vi "action.vi"(0 "HGF_FGV_Index":refnum<class "HGF_FGV_Index.lvclass">, 2 "Objects":refnum<class>[](array[class]), 5 "error in (no error)":errorcluster) -> (14 "dup HGF_FGV_Index":refnum<class "HGF_FGV_Index.lvclass">, 16 "dup Objects":refnum<class>[](array[class]), 19 "error out":errorcluster)   [LabVIEW 2012, in "HGF_FGV.lvlib" / "HGF_FGV_Index.lvclass"]
doc: "Return copy of addressed object from object array."
uses:
  HGF_FGV_Index.lvclass
  HGF_FGV_Index.lvclass/HGF_FGV_Index.ctl
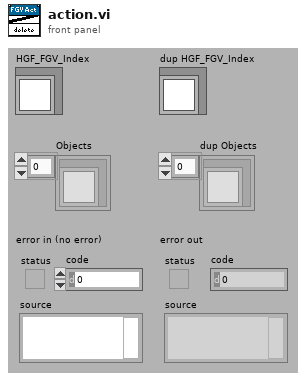
[diagram p1: front panel]
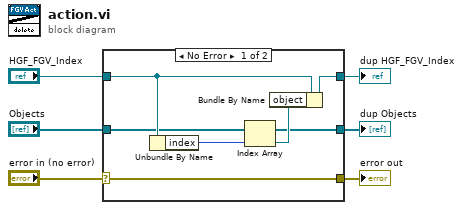
[diagram p0: block diagram]
diagram:
  n1 = case shown="No Error" "error in (no error)" {
    selector: "error in (no error)" -> [w12 w15]
    tunnel: [w12 w15] -> w5
    tunnel: [w11 w14] -> w3
    tunnel: "HGF_FGV_Index" -> [w10 w14]
    tunnel: [w7 w13] -> w2
    tunnel: "Objects" -> [w7 w13]
    frame No Error {
      n2 = Unbundle By Name(w10) -> ("index"=w8:u32)
      n3 = Index Array(array=w7, index=w8) -> (element=w9:refnum<class>)
      n4 = Bundle By Name(cluster=w10, "object"=w9) -> (w11:refnum<class "HGF_FGV_Index.lvclass">)
    }
    frame Error {
    }
  }
  "error out" <- w5
  "dup HGF_FGV_Index" <- w3
  "dup Objects" <- w2
